vi "Line_Send.vi"(9 "message":string, 10 "Key":string) -> ()   [LabVIEW 2019]
uses:
  <vilib>/httpClient/POSTBuffer.vi
  <vilib>/httpClient/LabVIEWHTTPClient.lvlib
  <vilib>/addons/Tools/Unicode/UTF8 Tools.lvlib
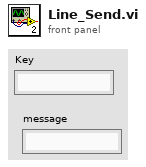
[diagram p1: front panel]
types:
  T1 = typedef "LabVIEWHTTPClient.lvlib/ClientHandle.ctl" = refnum<k1>
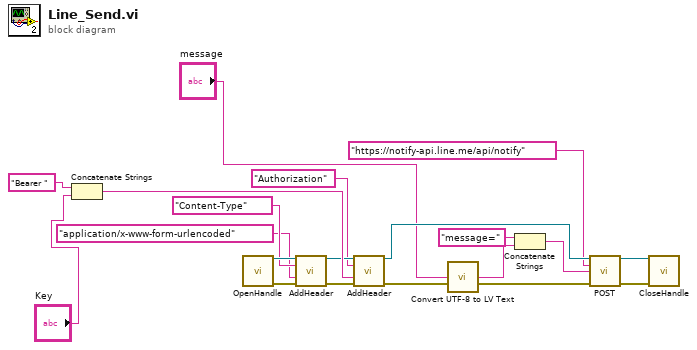
[diagram p0: block diagram]
diagram:
  n1 = Concatenate Strings("Bearer ", "Key") -> (w16:string)
  n2 = call <vilib>:"OpenHandle.vi"() -> ("client handle out"=w9:T1, "error out"=w10:errorcluster)  [unwired: 14 in]
  n3 = call <vilib>:"AddHeader.vi"("client handle"=w9, "header"="Content-Type", "value"="application/x-www-form-urlencoded", "error in (no error)"=w10) -> ("client handle out"=w12:T1, "error out"=w11:errorcluster)  [unwired: 10 in]
  n4 = call <vilib>:"AddHeader.vi"("client handle"=w12, "header"="Authorization", "value"=w16, "error in (no error)"=w11) -> ("client handle out"=w13:T1, "error out"=w17:errorcluster)  [unwired: 10 in]
  n5 = call <vilib>:"Convert UTF-8 to LV Text.vi"("UTF-8 Text"="message", "error in"=w17) -> ("LV Text"=w19:string, "error out"=w18:errorcluster)  [unwired: 12 in]
  n6 = Concatenate Strings("message=", w19) -> (w20:string)
  n7 = call-poly <vilib>:"POST.vi"("client handle"=w13, "url"="https://notify-api.line.me/api/notify", "buffer"=w20, "error in (no error)"=w18) -> ("client handle out"=w14:T1, "error out"=w15:errorcluster)  [unwired: 8 in, 2 out]
  n8 = call <vilib>:"CloseHandle.vi"("client handle"=w14, "error in (no error)"=w15) -> ()  [unwired: 13 in, 1 out]
